vi "benchmark.vi"() -> ()   [LabVIEW 2020]
uses:
  d590bb04-64b7-418b-b403-fb8384ec21ac.vi
  702f543a-3129-4d75-8bf4-3d8dadfbe18f.vi
  global/Global 1.vi
panel:
  out "log":string
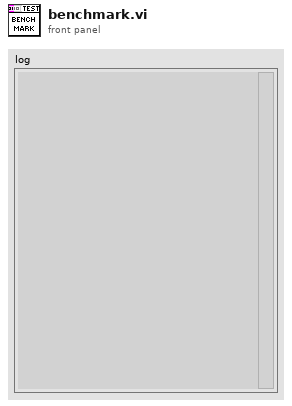
[diagram p1: front panel]
types:
  T1 = cluster{"ref":cluster{"DVR":refnum<data-value>, "Notif":refnum<notifier>}, "log":string, "read":u32, "write":u32, "write-toggle":u32}
  T2 = enum16{"init", "write", "write-toggle", "read", "log"}
  T3 = enum16{"Global", "DVR (FGV + MAP)", "DVR (FGV)", "DVR", "FGV", "Notif (FGV)", "Notif"}
  T4 = enum16{"Global", "DVR (FGV + MAP)", "DVR (FGV)", "DVR", "FGV", "Notif (FGV)", "Notif"}[]
  T5 = enum16{"init", "write", "write-toggle", "read", "log"}[]
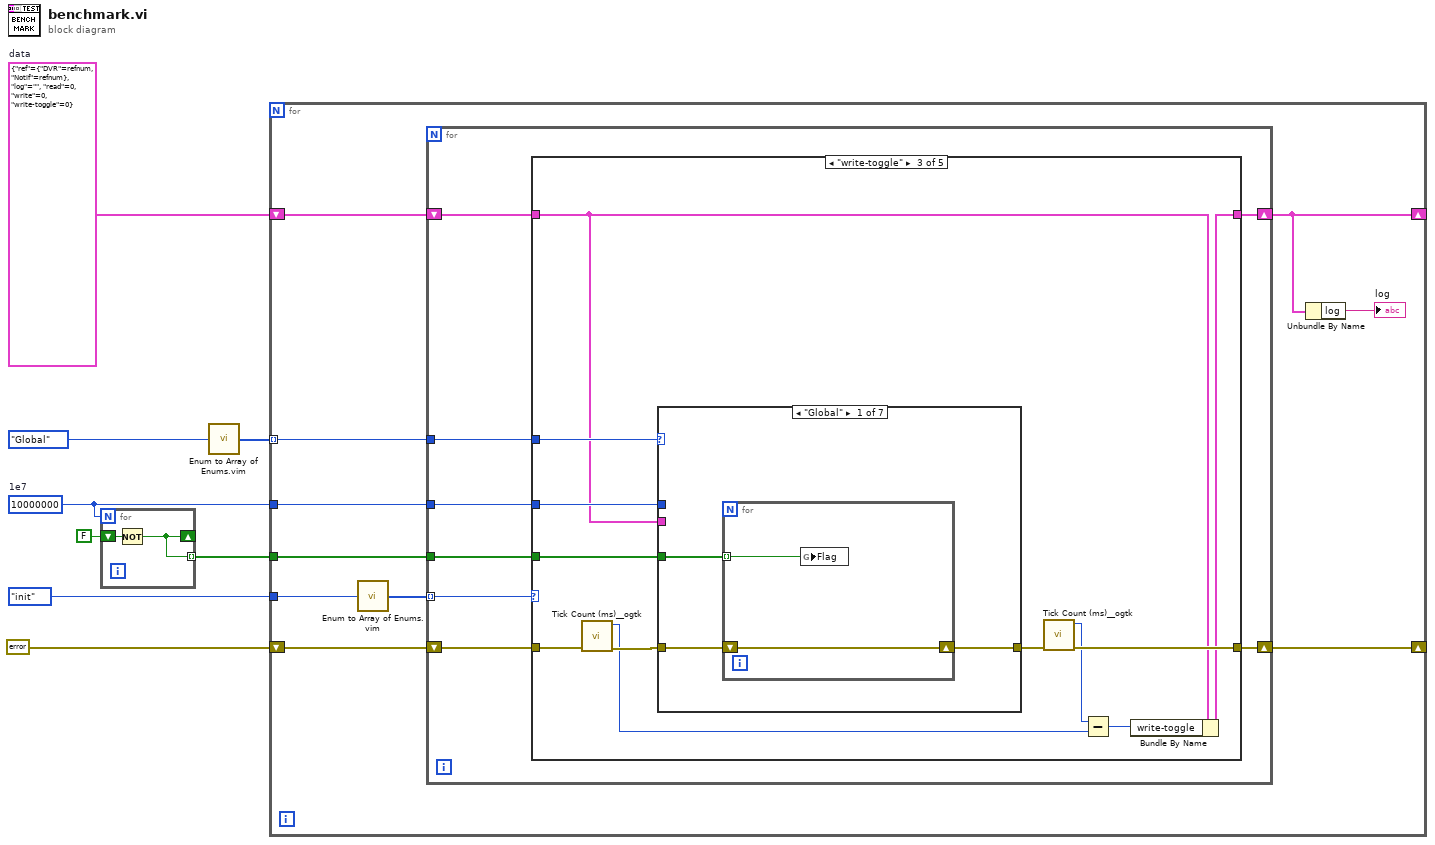
[diagram p0: block diagram]
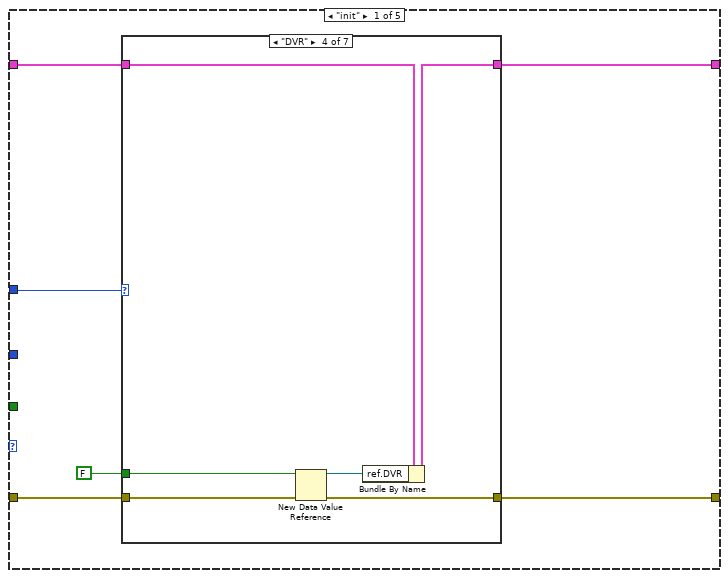
[diagram p2: hidden frame]
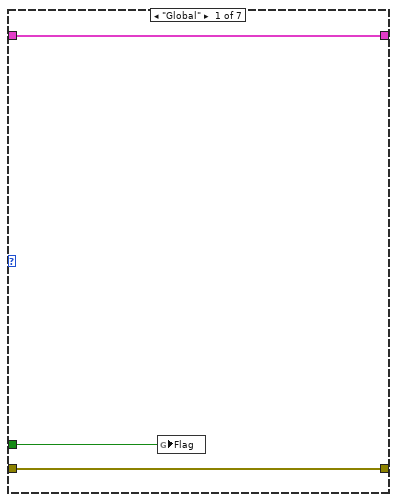
[diagram p3: hidden frame]
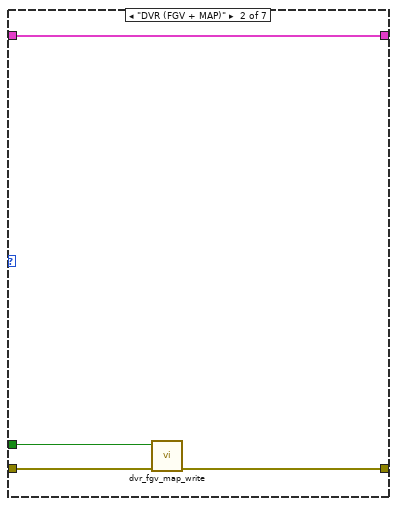
[diagram p4: hidden frame]
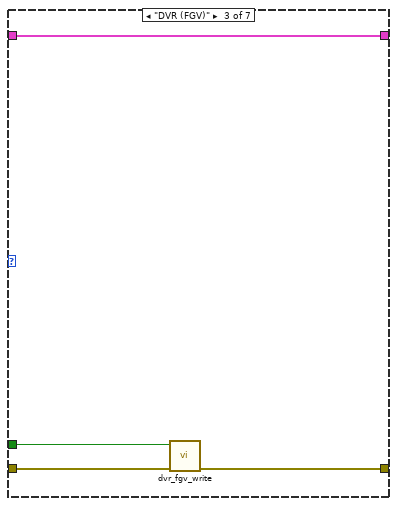
[diagram p5: hidden frame]
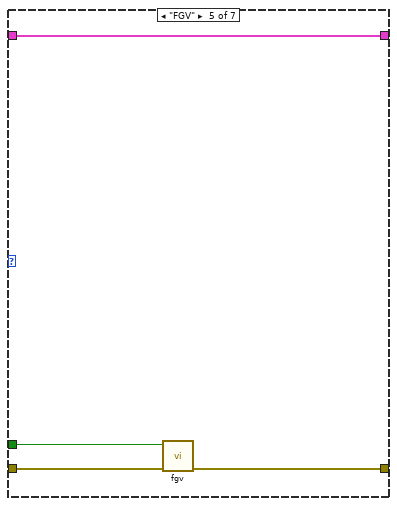
[diagram p6: hidden frame]
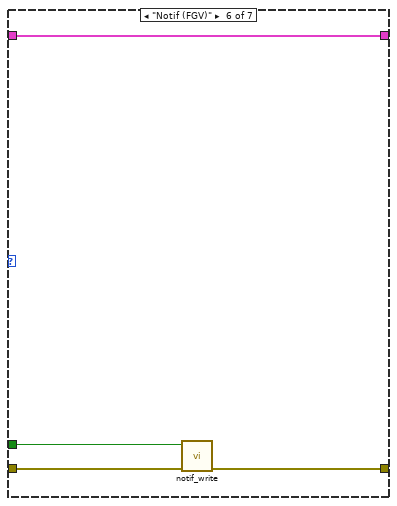
[diagram p7: hidden frame]
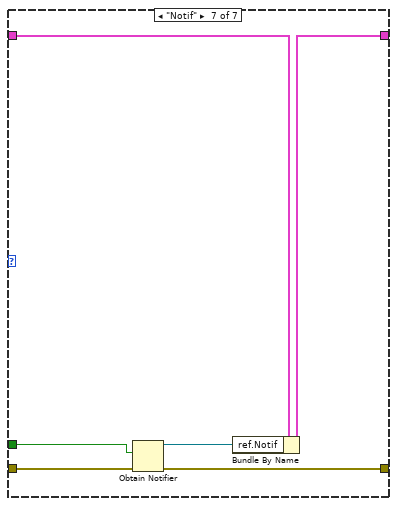
[diagram p8: hidden frame]
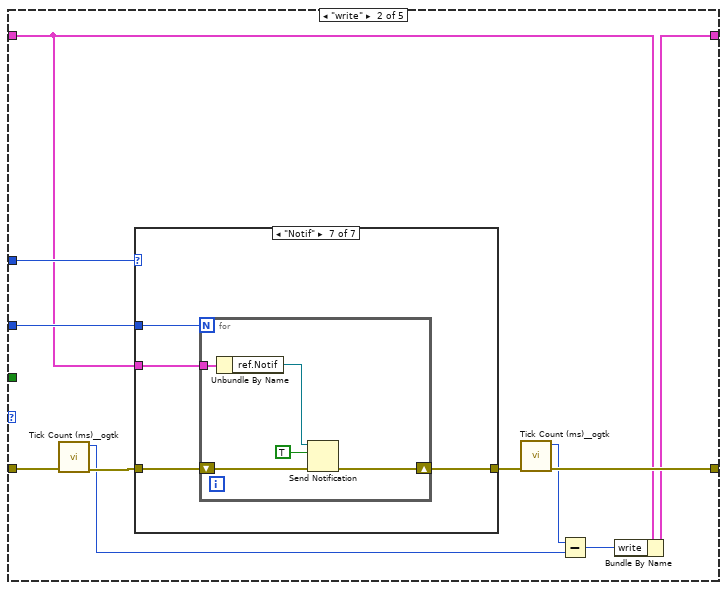
[diagram p9: hidden frame]
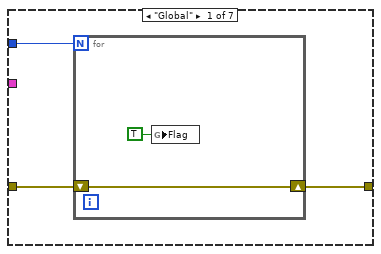
[diagram p10: hidden frame]
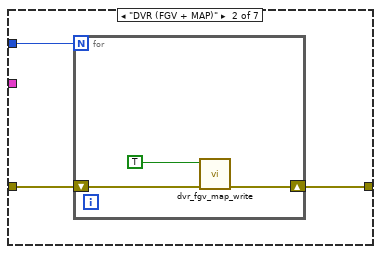
[diagram p11: hidden frame]
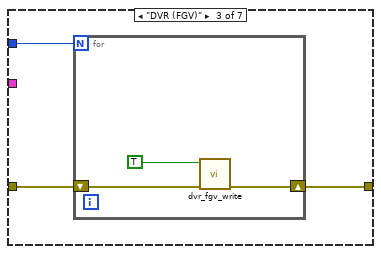
[diagram p12: hidden frame]
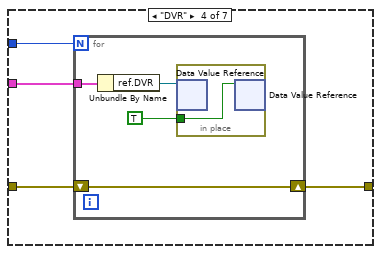
[diagram p13: hidden frame]
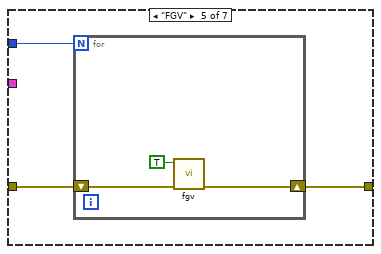
[diagram p14: hidden frame]
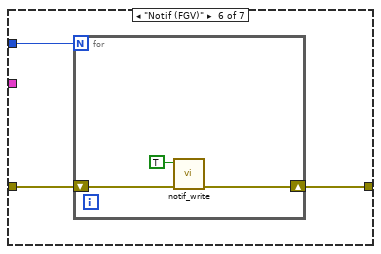
[diagram p15: hidden frame]
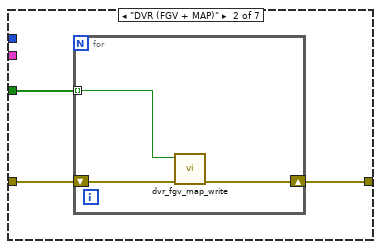
[diagram p16: hidden frame]
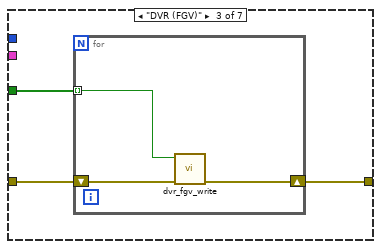
[diagram p17: hidden frame]
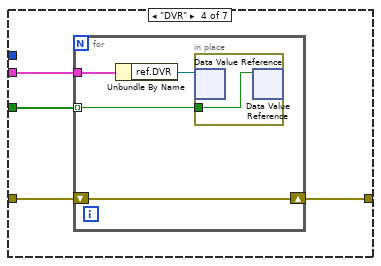
[diagram p18: hidden frame]
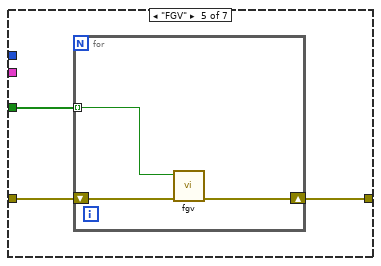
[diagram p19: hidden frame]
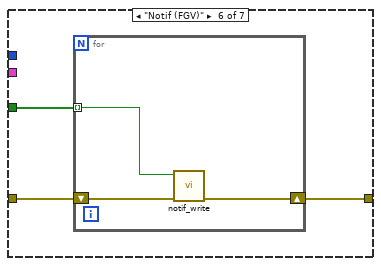
[diagram p20: hidden frame]
diagram:
  w1 = T1 {"ref"={"DVR"=refnum, "Notif"=refnum}, "log"="", "read"=0, "write"=0, "write-toggle"=0}  # data
  w4 = 10000000  # 1e7
  n1 = for {
    N: w4 -> [_]
    shift-right: [w9] -> _
    shift-left: FALSE -> [w10]
    tunnel: [w9] -> w2 mode=indexing
    n2 = Not(x=w10) -> (.not. x?=w9:bool)
  }
  n3 = call "Enum to Array of Enums.vim"("enum"=T3."Global") -> ("array of enums"=w6:T4)
  n4 = for {
    shift-right: [w18] -> _
    shift-left: errorcluster {"status"=FALSE, "code"=0, "source"=""} ("error constant") -> [w20]
    tunnel: w6 -> [w15] mode=indexing
    tunnel: T2."init" -> [w19]
    tunnel: w4 -> [w17]
    tunnel: w2 -> [w14]
    shift-right: [w11] -> _
    shift-left: w1 -> [w13]
    n5 = call "Enum to Array of Enums.vim"("enum"=w19) -> ("array of enums"=w16:T5)
    n6 = for {
      tunnel: w16 -> [w28] mode=indexing
      shift-right: [w24] -> w18
      shift-left: w20 -> [w25]
      tunnel: w17 -> [w27]
      tunnel: w15 -> [w26]
      tunnel: w14 -> [w23]
      shift-right: [w21] -> w11
      shift-left: w13 -> [w22]
      n7 = case shown="\"write-toggle\"" w28 {
        tunnel: w27 -> [_ w76 w135 w193 w236]
        tunnel: w26 -> [w34 w75 w134 w192 w238]
        tunnel: w25 -> [w33 w74 w133 w191 w239]
        tunnel: [w32 w71 w130 w188 w240] -> w24
        tunnel: w23 -> [_ _ w127 _ _]
        tunnel: w22 -> [w30 w68 w126 w185 w237]
        tunnel: [w29 w67 w125 w184 w241] -> w21
        frame "init" {
          n8 = case shown="\"DVR\"" w34 {
            tunnel: w33 -> [w37 w41 w44 w51 w54 w58 w64]
            tunnel: [w37 w40 w43 w50 w52 w57 w62] -> w32
            tunnel: FALSE ("Flag") -> [w36 w39 w45 w49 w53 w56 w63]
            tunnel: w30 -> [w35 w38 w42 w48 w55 w59 w65]
            tunnel: [w35 w38 w42 w47 w55 w59 w61] -> w29
            frame "Global" {
              n9 = global write "Global 1.vi" "Flag"(w36) -> ()
            }
            frame "DVR (FGV + MAP)" {
              n10 = call "dvr_fgv_map_write.vi"("error in (no error)"=w41, "value"=w39) -> ("error out"=w40:errorcluster)  [unwired: 9 in]
            }
            frame "DVR (FGV)" {
              n11 = call "dvr_fgv_write.vi"("error in (no error)"=w44, "Boolean"=w45) -> ("error out"=w43:errorcluster)  [unwired: 9 in]
            }
            frame "DVR" {
              n12 = New Data Value Reference(data value=w49, error in=w51) -> (data value reference=w46:refnum<data-value>, error out=w50:errorcluster)
              n13 = Bundle By Name(cluster=w48, "ref.DVR"=w46) -> (w47:T1)
            }
            frame "FGV" {
              n14 = call "fgv.vi"("error in (no error)"=w54, "Flag"=w53) -> ("error out"=w52:errorcluster)  [unwired: 8 in, 1 out]
            }
            frame "Notif (FGV)" {
              n15 = call "notif_write.vi"("error in (no error)"=w58, "notification"=w56) -> ("error out"=w57:errorcluster)  [unwired: 9 in]
            }
            frame "Notif" {
              n16 = Obtain Notifier(notification data type=w63, error in (no error)=w64) -> (notifier out=w60:refnum<notifier>, error out=w62:errorcluster)  [unwired: 2 in, 1 out]
              n17 = Bundle By Name(cluster=w65, "ref.Notif"=w60) -> (w61:T1)
            }
          }
        }
        frame "write" {
          n18 = call <userlib>:"Tick Count (ms)__ogtk.vi"("error in (no error)"=w74) -> ("error out"=w73:errorcluster, "millisecond timer value"=w70:u32)  [unwired: 9 in]
          n19 = case shown="\"Notif\"" w75 {
            tunnel: [w79 w84 w90 w97 w105 w111 w118] -> w72
            tunnel: w73 -> [w78 w83 w89 w96 w104 w110 w117]
            tunnel: w76 -> [w77 w82 w88 w95 w103 w109 w116]
            tunnel: w68 -> [_ _ _ w94 _ _ w115]
            frame "Global" {
              n20 = for {
                N: w77 -> [_]
                shift-right: [w80] -> w79
                shift-left: w78 -> [w80]
                n21 = global write "Global 1.vi" "Flag"(TRUE ("Flag")) -> ()
              }
            }
            frame "DVR (FGV + MAP)" {
              n22 = for {
                N: w82 -> [_]
                shift-right: [w85] -> w84
                shift-left: w83 -> [w86]
                n23 = call "dvr_fgv_map_write.vi"("error in (no error)"=w86, "value"=TRUE ("Flag")) -> ("error out"=w85:errorcluster)  [unwired: 9 in]
              }
            }
            frame "DVR (FGV)" {
              n24 = for {
                N: w88 -> [_]
                shift-right: [w91] -> w90
                shift-left: w89 -> [w92]
                n25 = call "dvr_fgv_write.vi"("error in (no error)"=w92, "Boolean"=TRUE ("Flag")) -> ("error out"=w91:errorcluster)  [unwired: 9 in]
              }
            }
            frame "DVR" {
              n26 = for {
                N: w95 -> [_]
                shift-right: [w101] -> w97
                shift-left: w96 -> [w101]
                tunnel: w94 -> [w100]
                n27 = Unbundle By Name(w100) -> ("ref.DVR"=w99:refnum<data-value>)
                n28 = in-place {
                  in-place-border: TRUE ("Flag") -> [w102]
                  n29 = in-place-dvr #1(w99) -> ()  [unwired: 2 out]
                  n30 = in-place-dvr #1(w102) -> ()  [unwired: 2 out]
                }
              }
            }
            frame "FGV" {
              n31 = for {
                N: w103 -> [_]
                shift-right: [w107] -> w105
                shift-left: w104 -> [w108]
                n32 = call "fgv.vi"("error in (no error)"=w108, "Flag"=TRUE) -> ("error out"=w107:errorcluster)  [unwired: 8 in, 1 out]
              }
            }
            frame "Notif (FGV)" {
              n33 = for {
                N: w109 -> [_]
                shift-right: [w113] -> w111
                shift-left: w110 -> [w114]
                n34 = call "notif_write.vi"("error in (no error)"=w114, "notification"=TRUE ("Flag")) -> ("error out"=w113:errorcluster)  [unwired: 9 in]
              }
            }
            frame "Notif" {
              n35 = for {
                N: w116 -> [_]
                shift-right: [w122] -> w118
                shift-left: w117 -> [w123]
                tunnel: w115 -> [w120]
                n36 = Unbundle By Name(w120) -> ("ref.Notif"=w119:refnum<notifier>)
                n37 = Send Notification(notification=TRUE ("Flag"), notifier=w119, error in (no error)=w123) -> (error out=w122:errorcluster)  [unwired: 1 out]
              }
            }
          }
          n38 = call <userlib>:"Tick Count (ms)__ogtk.vi"("error in (no error)"=w72) -> ("error out"=w71:errorcluster, "millisecond timer value"=w69:u32)  [unwired: 9 in]
          n39 = Subtract(x=w69, y=w70) -> (x-y=w66:u32)
          n40 = Bundle By Name(cluster=w68, "write"=w66) -> (w67:T1)
        }
        frame "write-toggle" {
          n41 = call <userlib>:"Tick Count (ms)__ogtk.vi"("error in (no error)"=w133) -> ("error out"=w132:errorcluster, "millisecond timer value"=w129:u32)  [unwired: 9 in]
          n42 = case shown="\"Global\"" w134 {
            tunnel: [w138 w143 w149 w156 w164 w170 w177] -> w131
            tunnel: w132 -> [w137 w142 w148 w155 w163 w169 w176]
            tunnel: w135 -> [_ _ _ _ _ _ _]
            tunnel: w127 -> [w136 w141 w147 w154 w162 w168 w175]
            tunnel: w126 -> [_ _ _ w153 _ _ w174]
            frame "Global" {
              n43 = for {
                shift-right: [w140] -> w138
                shift-left: w137 -> [w140]
                tunnel: w136 -> [w139] mode=indexing
                n44 = global write "Global 1.vi" "Flag"(w139) -> ()
              }
            }
            frame "DVR (FGV + MAP)" {
              n45 = for {
                shift-right: [w144] -> w143
                shift-left: w142 -> [w145]
                tunnel: w141 -> [w146] mode=indexing
                n46 = call "dvr_fgv_map_write.vi"("error in (no error)"=w145, "value"=w146) -> ("error out"=w144:errorcluster)  [unwired: 9 in]
              }
            }
            frame "DVR (FGV)" {
              n47 = for {
                shift-right: [w150] -> w149
                shift-left: w148 -> [w151]
                tunnel: w147 -> [w152] mode=indexing
                n48 = call "dvr_fgv_write.vi"("error in (no error)"=w151, "Boolean"=w152) -> ("error out"=w150:errorcluster)  [unwired: 9 in]
              }
            }
            frame "DVR" {
              n49 = for {
                shift-right: [w160] -> w156
                shift-left: w155 -> [w160]
                tunnel: w154 -> [w157] mode=indexing
                tunnel: w153 -> [w158]
                n50 = Unbundle By Name(w158) -> ("ref.DVR"=w159:refnum<data-value>)
                n51 = in-place {
                  in-place-border: w157 -> [w161]
                  n52 = in-place-dvr #2(w159) -> ()  [unwired: 2 out]
                  n53 = in-place-dvr #2(w161) -> ()  [unwired: 2 out]
                }
              }
            }
            frame "FGV" {
              n54 = for {
                shift-right: [w166] -> w164
                shift-left: w163 -> [w167]
                tunnel: w162 -> [w165] mode=indexing
                n55 = call "fgv.vi"("error in (no error)"=w167, "Flag"=w165) -> ("error out"=w166:errorcluster)  [unwired: 8 in, 1 out]
              }
            }
            frame "Notif (FGV)" {
              n56 = for {
                shift-right: [w172] -> w170
                shift-left: w169 -> [w173]
                tunnel: w168 -> [w171] mode=indexing
                n57 = call "notif_write.vi"("error in (no error)"=w173, "notification"=w171) -> ("error out"=w172:errorcluster)  [unwired: 9 in]
              }
            }
            frame "Notif" {
              n58 = for {
                shift-right: [w178] -> w177
                shift-left: w176 -> [w179]
                tunnel: w175 -> [w180] mode=indexing
                tunnel: w174 -> [w181]
                n59 = Unbundle By Name(w181) -> ("ref.Notif"=w182:refnum<notifier>)
                n60 = Send Notification(notification=w180, notifier=w182, error in (no error)=w179) -> (error out=w178:errorcluster)  [unwired: 1 out]
              }
            }
          }
          n61 = call <userlib>:"Tick Count (ms)__ogtk.vi"("error in (no error)"=w131) -> ("error out"=w130:errorcluster, "millisecond timer value"=w128:u32)  [unwired: 9 in]
          n62 = Subtract(x=w128, y=w129) -> (x-y=w124:u32)
          n63 = Bundle By Name(cluster=w126, "write-toggle"=w124) -> (w125:T1)
        }
        frame "read" {
          n64 = call <userlib>:"Tick Count (ms)__ogtk.vi"("error in (no error)"=w191) -> ("error out"=w190:errorcluster, "millisecond timer value"=w187:u32)  [unwired: 9 in]
          n65 = case shown="\"FGV\"" w192 {
            tunnel: [w196 w201 w206 w212 w219 w225 w231] -> w189
            tunnel: w190 -> [w195 w200 w205 w211 w218 w224 w230]
            tunnel: w193 -> [w194 w199 w204 w210 w217 w223 w229]
            tunnel: w185 -> [_ _ _ w209 _ _ w228]
            frame "Global" {
              n66 = for {
                N: w194 -> [_]
                shift-right: [w198] -> w196
                shift-left: w195 -> [w198]
                n67 = global read "Global 1.vi" "Flag"() -> (w197:bool)
                n68 = Not(x=w197) -> ()  [unwired: 1 out]
              }
            }
            frame "DVR (FGV + MAP)" {
              n69 = for {
                N: w199 -> [_]
                shift-right: [w202] -> w201
                shift-left: w200 -> [w203]
                n70 = call "dvr_fgv_map_read.vi"("error in (no error)"=w203) -> ("error out"=w202:errorcluster)  [unwired: 9 in, 1 out]
              }
            }
            frame "DVR (FGV)" {
              n71 = for {
                N: w204 -> [_]
                shift-right: [w207] -> w206
                shift-left: w205 -> [w208]
                n72 = call "dvr_fgv_read.vi"("error in (no error)"=w208) -> ("error out"=w207:errorcluster)  [unwired: 9 in, 1 out]
              }
            }
            frame "DVR" {
              n73 = for {
                N: w210 -> [_]
                shift-right: [w215] -> w212
                shift-left: w211 -> [w215]
                tunnel: w209 -> [w213]
                n74 = Unbundle By Name(w213) -> ("ref.DVR"=w214:refnum<data-value>)
                n75 = in-place {
                  in-place-border: [w216] -> _
                  n76 = in-place-dvr #3(w214) -> (w216:bool)  [unwired: 1 out]
                  n77 = in-place-dvr #3(w216) -> ()  [unwired: 2 out]
                }
              }
            }
            frame "FGV" {
              n78 = for {
                N: w217 -> [_]
                shift-right: [w221] -> w219
                shift-left: w218 -> [w222]
                n79 = call "fgv.vi"("error in (no error)"=w222, "R/W (Write = True)"=FALSE) -> ("error out"=w221:errorcluster)  [unwired: 8 in, 1 out]
              }
            }
            frame "Notif (FGV)" {
              n80 = for {
                N: w223 -> [_]
                shift-right: [w226] -> w225
                shift-left: w224 -> [w227]
                n81 = call "notif_read.vi"("error in (no error)"=w227) -> ("error out"=w226:errorcluster)  [unwired: 9 in, 1 out]
              }
            }
            frame "Notif" {
              n82 = for {
                N: w229 -> [_]
                shift-right: [w234] -> w231
                shift-left: w230 -> [w235]
                tunnel: w228 -> [w233]
                n83 = Unbundle By Name(w233) -> ("ref.Notif"=w232:refnum<notifier>)
                n84 = Get Notifier Status(notifier=w232, error in (no error)=w235) -> (error out=w234:errorcluster)  [unwired: 4 out]
              }
            }
          }
          n85 = call <userlib>:"Tick Count (ms)__ogtk.vi"("error in (no error)"=w189) -> ("error out"=w188:errorcluster, "millisecond timer value"=w186:u32)  [unwired: 9 in]
          n86 = Subtract(x=w186, y=w187) -> (x-y=w183:u32)
          n87 = Bundle By Name(cluster=w185, "read"=w183) -> (w184:T1)
        }
        frame "log" {
          n88 = in-place {
            in-place-border: [w255] -> w240
            in-place-border: w239 -> [w258]
            in-place-border: w238 -> [w252]
            in-place-border: w237 -> [w251]
            in-place-border: w236 -> [w246]
            n89 = in-place-cluster #4(w237) -> ("log"=w257:string)
            n90 = Unbundle By Name(w251) -> ("write"=w250:u32, "write-toggle"=w249:u32, "read"=w248:u32)
            n91 = Build Array(w250, w249, w248) -> (w247:u32[])
            n92 = for {
              tunnel: w247 -> [w263] mode=indexing
              tunnel: w246 -> [w262]
              tunnel: [w259] -> w245 mode=indexing
              n93 = Divide(x=w263, y=w262) -> (x/y=w261:dbl)
              n94 = Multiply(x=w261, y=1000000.0) -> (x*y=w259:dbl)
            }
            n95 = Index Array(array=w245) -> (element #1=w244:dbl, element #2=w243:dbl, element #3=w242:dbl)  [unwired: 3 in]
            n96 = Format Into String(format string="Current step: %s\nwrite: %d [ns]\nwrite-toggle: %d [ns]\nread: %d [ns]\n---------------------\n", error in=w258, w252, w244, w243, w242) -> (resulting string=w253:string, error out=w255:errorcluster)  [unwired: 1 in]
            n97 = Concatenate Strings(w257, w253) -> (w256:string)
            n98 = in-place-cluster #4("log"=w256) -> (w241:T1)
          }
        }
      }
    }
    n99 = Unbundle By Name(w11) -> ("log"=→"log":string)
  }
